vi "CalculateDistances.vi"(10 "Centroids2":dbl[][](array[numeric])=[[305.5627746582031, 67.89103698730469], [341.9431457519531, 72.40214538574219], [232.1138153076172, 91.70089721679688], [411.30303955078125, 99.19172668457031], [201.31768798828125, 112.402099609375], [178.73162841796875, 140.29721069335938], [455.8645935058594, 155.0275421142578], [163.60015869140625, 176.1148223876953], [154.8563995361328, 211.54965209960938], [476.7146911621094, 222.72250366210938], [37.367530822753906, 236.38706970214844], [157.02395629882812, 249.5926971435547], [167.57664489746094, 281.2937927246094], [460.26348876953125, 297.98388671875], [184.57943725585938, 313.2145690917969], [442.5791320800781, 331.2660827636719], [206.3518829345703, 345.27783203125], [415.7437438964844, 355.53765869140625], [239.37156677246094, 369.4365539550781], [382.6512451171875, 372.81396484375], [268.6066589355469, 375.957275390625], [345.42205810546875, 383.692626953125], [307.2210388183594, 390.125], [315.5556335449219, 454.518798828125], [261.72613525390625, 461.53814697265625], [399.8280944824219, 466.7994079589844], [450.890869140625, 478.2618103027344]], 11 "Centroids1":dbl[][](array[numeric])=[[305.5627746582031, 67.89103698730469], [341.9431457519531, 72.40214538574219], [232.1138153076172, 91.70089721679688], [411.30303955078125, 99.19172668457031], [201.31768798828125, 112.402099609375], [178.73162841796875, 140.29721069335938], [455.8645935058594, 155.0275421142578], [163.60015869140625, 176.1148223876953], [154.8563995361328, 211.54965209960938], [476.7146911621094, 222.72250366210938], [37.367530822753906, 236.38706970214844], [157.02395629882812, 249.5926971435547], [167.57664489746094, 281.2937927246094], [460.26348876953125, 297.98388671875], [184.57943725585938, 313.2145690917969], [442.5791320800781, 331.2660827636719], [206.3518829345703, 345.27783203125], [415.7437438964844, 355.53765869140625], [239.37156677246094, 369.4365539550781], [382.6512451171875, 372.81396484375], [268.6066589355469, 375.957275390625], [345.42205810546875, 383.692626953125], [307.2210388183594, 390.125], [315.5556335449219, 454.518798828125], [261.72613525390625, 461.53814697265625], [399.8280944824219, 466.7994079589844], [450.890869140625, 478.2618103027344]]) -> (3 "Distances":dbl[][](array[numeric]))   [LabVIEW 2017, in "ImageAcquisitionLibrary.lvlib"]
uses:
  ImageAcquisitionLibrary.lvlib
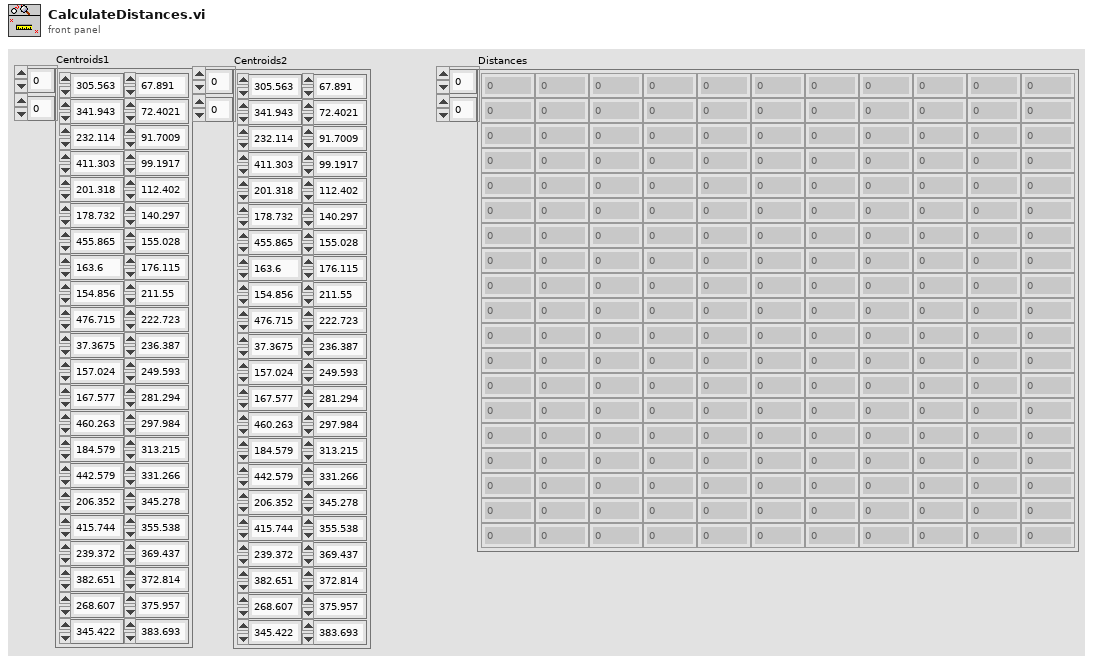
[diagram p1: front panel]
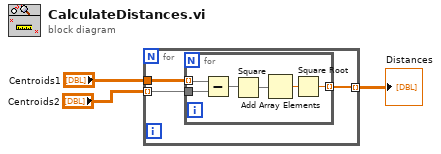
[diagram p0: block diagram]
diagram:
  n1 = for {
    tunnel: "Centroids2" -> [w5] mode=indexing
    tunnel: "Centroids1" -> [w6]
    tunnel: [w4] -> w1 mode=indexing
    n2 = for {
      tunnel: w6 -> [w11] mode=indexing
      tunnel: w5 -> [w12]
      tunnel: [w7] -> w4 mode=indexing
      n3 = Subtract(x=w11, y=w12) -> (x-y=w10:dbl[])
      n4 = Square(x=w10) -> (x^2=w9:dbl[])
      n5 = Add Array Elements(numeric array=w9) -> (sum=w8:dbl)
      n6 = Square Root(x=w8) -> (sqrt(x)=w7:dbl)
    }
  }
  "Distances" <- w1
